vi "WordToHex.vi"(11 "WORD":u16[](array[numeric])) -> (3 "数组":u16[](array[numeric]) format="%04xH")   [LabVIEW 2016, in "总磷.lvlib"]
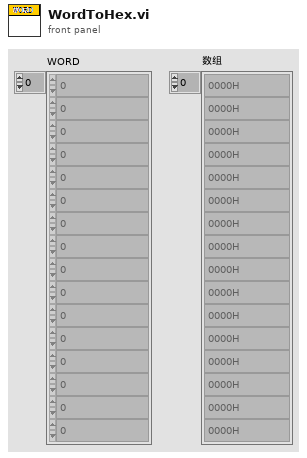
[diagram p1: front panel]
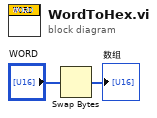
[diagram p0: block diagram]
diagram:
  n1 = Swap Bytes(anything="WORD") -> (byte swapped=→"数组":u16[])
